vi "CLASS - 2DSortData.vi"(7 "Index":cluster{"X":i32, "Y":i32}, 8 "error in":errorcluster, 10 "Y":dbl[](array[numeric]), 11 "X":dbl[][](array[numeric])) -> (0 "error out":errorcluster, 3 "Array":cluster{"Array":dbl[], "Array":dbl[]}[](array[cluster]))   [LabVIEW 2020]
doc: "Rearrange the Train data"
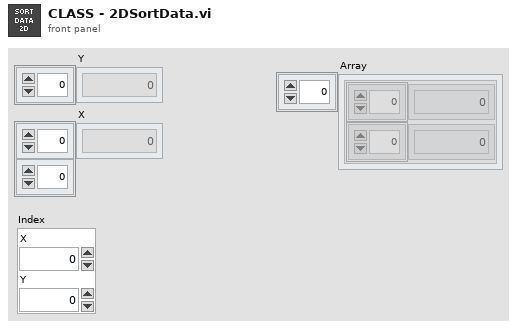
[diagram p1: front panel]
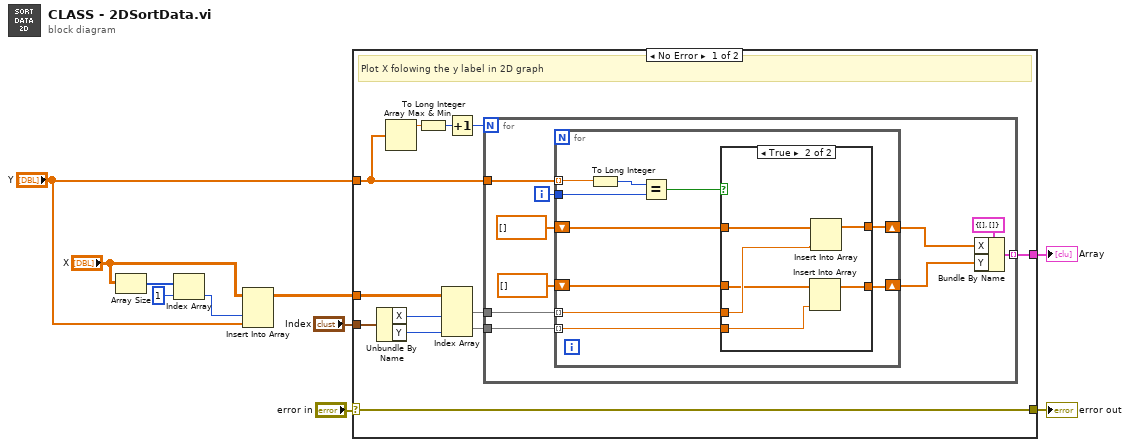
[diagram p0: block diagram]
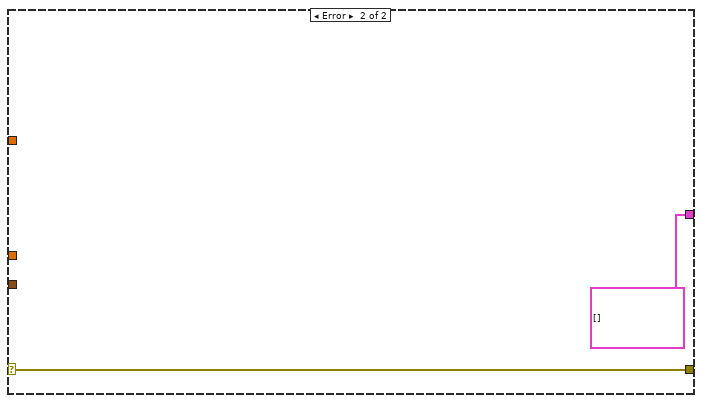
[diagram p3: hidden frame]
diagram:
  n1 = Array Size(array="X") -> (size(s)=w3:i32[])
  n2 = Index Array(array=w3, index=1) -> (element=w1:i32)
  n3 = Insert Into Array(array="X", index (col)=w1, new element="Y") -> (w6:dbl[][])  [unwired: 1 in]
  n4 = case shown="No Error" "error in" {
    selector: "error in" -> [w20 w52]
    tunnel: w6 -> [w14 _]
    tunnel: "Y" -> [w16 _]
    tunnel: [w20 w52] -> w7
    tunnel: [w19 cluster{dbl[], dbl[]}[] []] -> w9
    tunnel: "Index" -> [w13 _]
    frame No Error {
      # "Plot X folowing the y label in 2D graph"
      n5 = Unbundle By Name(w13) -> ("X"=w12:i32, "Y"=w11:i32)
      n6 = Array Max & Min(array=w16) -> (max value=w18:dbl)  [unwired: 3 out]
      n7 = To Long Integer(number=w18) -> (32bit integer=w17:i32)
      n8 = Index Array(array=w14, index (col) #1=w12, index (col) #2=w11) -> (element #1=w22:dbl[], element #2=w21:dbl[])  [unwired: 2 in]
      n9 = Increment(x=w17) -> (x+1=w15:i32)
      n10 = for {
        N: w15 -> [_]
        tunnel: w22 -> [w32]
        tunnel: w21 -> [w31]
        tunnel: w16 -> [w30]
        tunnel: [w25] -> w19 mode=indexing
        i -> [w29]
        n11 = for {
          tunnel: w30 -> [w42] mode=indexing
          tunnel: w32 -> [w39] mode=indexing
          tunnel: w31 -> [w38] mode=indexing
          shift-right: [w36] -> w24
          shift-left: dbl[] [] -> [w35]
          shift-right: [w37] -> w23
          shift-left: dbl[] [] -> [w34]
          tunnel: w29 -> [w33]
          n12 = To Long Integer(number=w42) -> (32bit integer=w41:i32)
          n13 = Equal?(x=w41, y=w33) -> (x = y?=w40:bool)
          n14 = case shown="True" w40 {
            tunnel: w39 -> [_ w49]
            tunnel: w38 -> [_ w45]
            tunnel: [w43 w47] -> w37
            tunnel: [w44 w48] -> w36
            tunnel: w35 -> [w44 w50]
            tunnel: w34 -> [w43 w46]
            frame False {
            }
            frame True {
              n15 = Insert Into Array(array=w46, new element=w45) -> (w47:dbl[])  [unwired: 1 in]
              n16 = Insert Into Array(array=w50, new element=w49) -> (w48:dbl[])  [unwired: 1 in]
            }
          }
        }
        n17 = Bundle By Name(cluster=cluster{"X":dbl[], "Y":dbl[]} {"X"=[], "Y"=[]} ("output cluster"), "X"=w24, "Y"=w23) -> (w25:cluster{"X":dbl[], "Y":dbl[]})
      }
    }
    frame Error {
    }
  }
  "Array" <- w9
  "error out" <- w7
